vi "batch action wait on all.vi"() -> ()   [LabVIEW 2013]
uses:
  result/result.lvclass
  standard tasks/batch task/reporting type.ctl
  result/result.lvclass/result.ctl
  result/get data.vi
  result/get error.vi
  result/get owning task.vi
  result/get subresults.vi
  dispatcher/thread pool.lvclass
  standard reporters/event reporter/event reporter.lvclass
  standard tasks/batch task/batch task.lvclass
  standard action/wait action/wait action.lvclass
panel:
  out "owning task":string
  out "error":errorcluster
  out "data":variant
  out "accessors:subresults":refnum<class "result.lvclass">[][](array[class])
  out "owning task":string[](array[string])
  out "Array 2":errorcluster[](array[cluster])
  out "Array":variant[](array[variant])
  out "Time":u32
  out "result":refnum<class "result.lvclass">
  out "error out":errorcluster
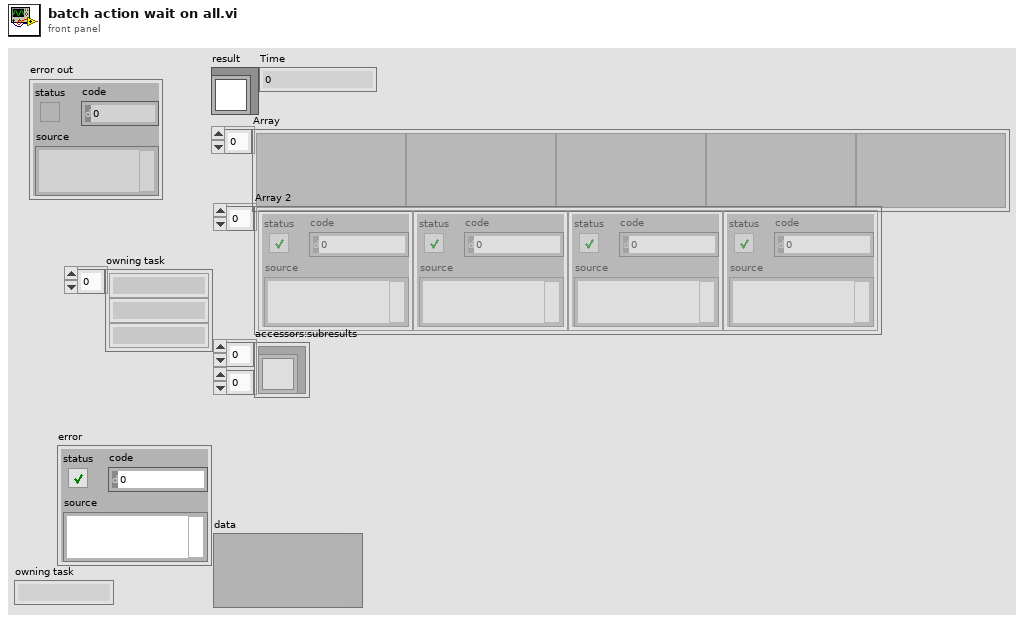
[diagram p1: front panel]
types:
  T1 = typedef "batch task.lvclass/reporting type.ctl" = enum16{"return immediately", "wait on all"}
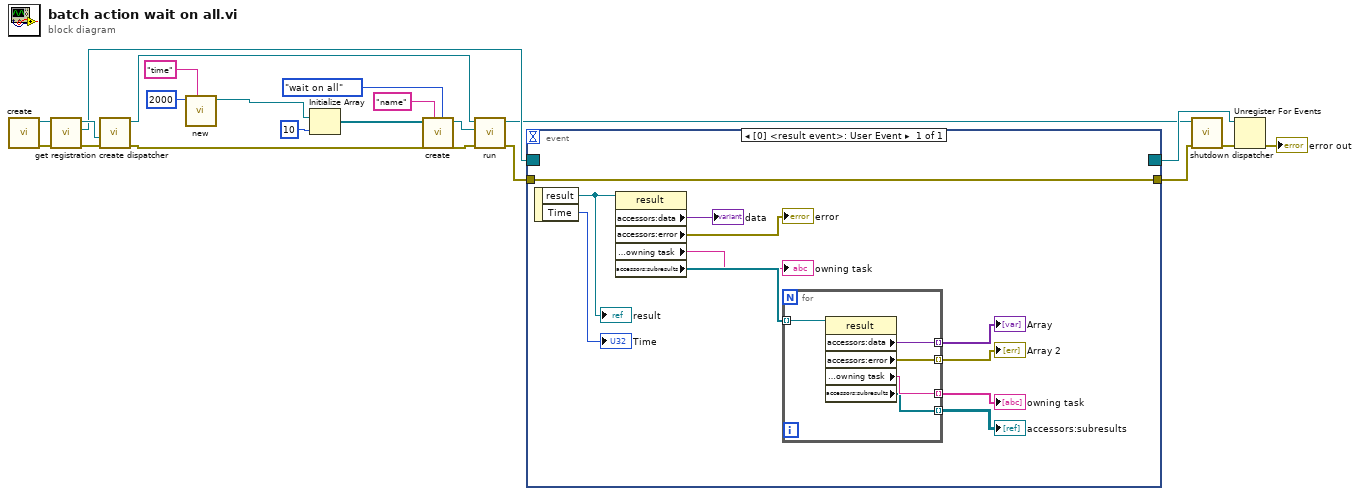
[diagram p0: block diagram]
diagram:
  n1 = call "create.vi"() -> ("error out"=w18:errorcluster, "event reporter out"=w19:refnum<class "event reporter.lvclass">)  [unwired: 10 in]
  n2 = call "get registration.vi"("error in"=w18, "event reporter in"=w19) -> ("error out"=w16:errorcluster, "result registration"=w15:refnum<event-registration>, "event reporter out"=w17:refnum<class "event reporter.lvclass">)  [unwired: 7 in]
  n3 = call "create dispatcher.vi"("error in"=w16, "default reporter"=w17) -> ("error out"=w20:errorcluster, "dispatcher"=w21:refnum<data-value>)  [unwired: 8 in]
  n4 = call "new.vi"("ID"="time", "timer"=2000) -> ("wait action out"=w3:refnum<class "wait action.lvclass">)  [unwired: 9 in]
  n5 = Initialize Array(w3, 10 ("dimension size")) -> (w7:refnum<class "wait action.lvclass">[])
  n6 = call "create.vi"("reporting type"=reporting_type."wait on all", "ID"="name", "tasks"=w7) -> ("batch task out"=w6:refnum<class "batch task.lvclass">)  [unwired: 8 in]
  n7 = call "run.vi"("error in"=w20, "task"=w6, "dispatcher"=w21) -> ("error out"=w9:errorcluster, "dispatcher out"=w13:refnum<data-value>)  [unwired: 7 in]
  n8 = event shown="[0] <result event>: User Event" {
    selector: w15 -> [_]
    dyn-events: [_] -> w14
    timeout: _ -> [_]
    tunnel: [w31] -> w10
    tunnel: w9 -> [w31]
    event User Event {
      n9 = event-data() -> ("result"=w30:refnum<class "result.lvclass">, "Time"=→"Time":u32)  [unwired: 1 in]
      "result" <- w30
      n10 = property class="result"(reference=w30) -> ("accessors:data"=→"data":variant, "accessors:error"=→"error":errorcluster, "accessors:owning task"=→"owning task":string, "accessors:subresults"=w29:refnum<class "result.lvclass">[])  [unwired: 1 in, 2 out]
      n11 = for {
        tunnel: w29 -> [w37] mode=indexing
        tunnel: [w36] -> w28 mode=indexing
        tunnel: [w35] -> w27 mode=indexing
        tunnel: [w34] -> w26 mode=indexing
        tunnel: [w33] -> w25 mode=indexing
        n12 = property class="result"(reference=w37) -> ("accessors:data"=w36:variant, "accessors:error"=w35:errorcluster, "accessors:owning task"=w34:string, "accessors:subresults"=w33:refnum<class "result.lvclass">[])  [unwired: 1 in, 2 out]
      }
      "Array" <- w28
      "Array 2" <- w27
      "owning task" <- w26
      "accessors:subresults" <- w25
    }
  }
  n13 = call "shutdown dispatcher.vi"("error in"=w10, "dispatcher"=w13) -> ("error out"=w12:errorcluster)  [unwired: 9 in]
  n14 = Unregister For Events(event registration refnum=w14, error in=w12) -> (error out=→"error out":errorcluster)
